vi "Task_04.vi"() -> ()   [LabVIEW 2015]
panel:
  out "Dict array 2":dbl[][](array[numeric])
  out "Dict array 1":dbl[][](array[numeric])
  out "3-8 in Array 2":i32
  out "3-8 in Array 1":i32
  out "Matching positions idnecies":i32[](array[numeric])
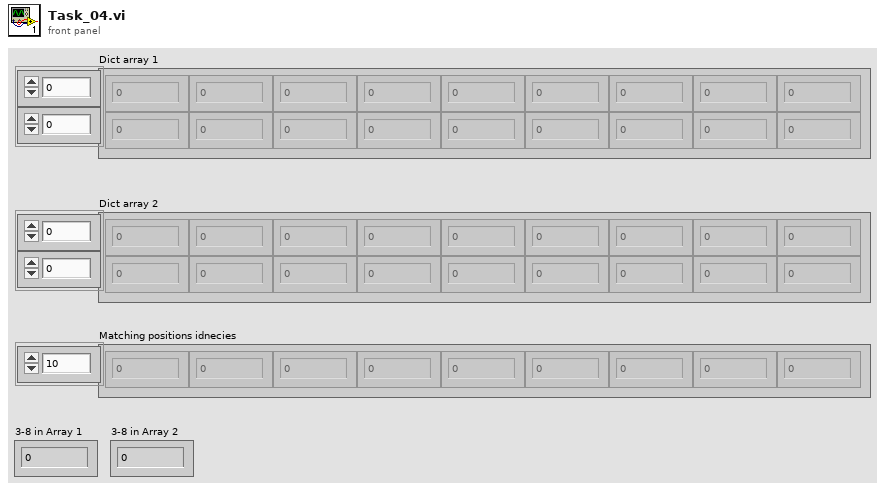
[diagram p1: front panel]
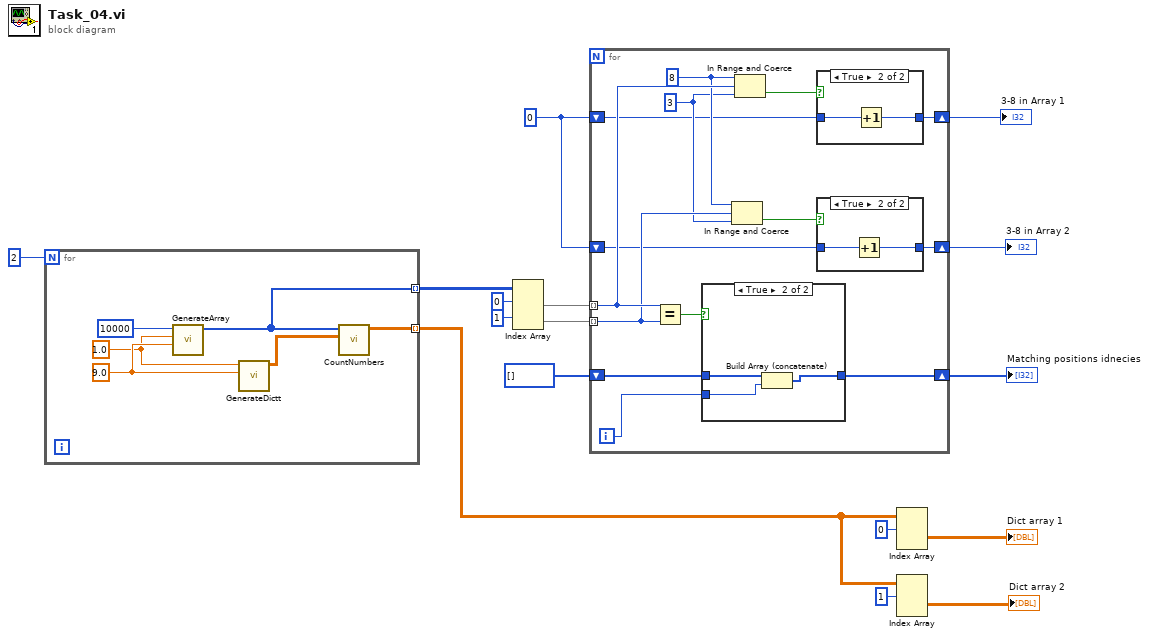
[diagram p0: block diagram]
diagram:
  w8 = 0
  n1 = for {
    N: 2 -> [_]
    tunnel: [w18] -> w15 mode=indexing
    tunnel: [w17] -> w4 mode=indexing
    w21 = 9.0 ("Stop")
    w20 = 1.0 ("Start")
    n2 = call "GenerateArray.vi"("Stop"=w21, "Start"=w20, "Array_size"=10000) -> ("Array"=w18:u8[])  [unwired: 8 in]
    n3 = call "GenerateDictt.vi"("Stop"=w21, "Start"=w20) -> ("Array"=w19:dbl[][])  [unwired: 9 in]
    n4 = call "CountNumbers.vi"("Array in"=w19, "Array 3"=w18) -> ("Array out"=w17:dbl[][])  [unwired: 9 in]
  }
  n5 = Index Array(array=w15, index (row) #1=0 ("index (row)"), index (row) #2=1 ("index (row)")) -> (element #1=w12:u8[], element #2=w11:u8[])  [unwired: 2 in]
  n6 = for {
    tunnel: w12 -> [w32] mode=indexing
    tunnel: w11 -> [w31] mode=indexing
    shift-right: [w33] -> w9
    shift-left: i32[] [] -> [w35]
    shift-right: [w25] -> w7
    shift-left: w8 -> [w26]
    shift-right: [w23] -> w6
    shift-left: w8 -> [w24]
    i -> [w34]
    w29 = u8 3 ("upper limit")
    w30 = u8 8 ("upper limit")
    n7 = Equal?(x=w32, y=w31) -> (x = y?=w36:bool)
    n8 = case shown="True" w36 {
      tunnel: w35 -> [w43 w46]
      tunnel: w34 -> [_ w45]
      tunnel: [w43 w44] -> w33
      frame False {
      }
      frame True {
        n9 = Build Array (concatenate)(w46, w45) -> (w44:i32[])
      }
    }
    n10 = In Range and Coerce(upper limit=w30, x=w31, lower limit=w29) -> (In Range?=w27:bool)  [unwired: 1 out]
    n11 = In Range and Coerce(upper limit=w30, x=w32, lower limit=w29) -> (In Range?=w28:bool)  [unwired: 1 out]
    n12 = case shown="True" w28 {
      tunnel: w26 -> [w40 w42]
      tunnel: [w40 w41] -> w25
      frame False {
      }
      frame True {
        n13 = Increment(x=w42) -> (x+1=w41:i32)
      }
    }
    n14 = case shown="True" w27 {
      tunnel: w24 -> [w37 w39]
      tunnel: [w37 w38] -> w23
      frame False {
      }
      frame True {
        n15 = Increment(x=w39) -> (x+1=w38:i32)
      }
    }
  }
  "Matching positions idnecies" <- w9
  "3-8 in Array 1" <- w7
  "3-8 in Array 2" <- w6
  n16 = Index Array(array=w4, index (dim 0)=0 ("index (page)")) -> (element=→"Dict array 1":dbl[][])  [unwired: 2 in]
  n17 = Index Array(array=w4, index (dim 0)=1 ("index (page)")) -> (element=→"Dict array 2":dbl[][])  [unwired: 2 in]
